vi "1 - Get XY and start end.vi"() -> ()   [LabVIEW 2013]
uses:
  <vilib>/vision/NI_Vision_Development_Module.lvlib
panel:
  out "appended array":dbl[](array[numeric])
  out "frame number XY top XY bottom":dbl[][](array[numeric])
  in  "fast forward":bool
  out "start":i32[](array[numeric])
  out "end":i32[](array[numeric])
  out "end":i32[](array[numeric])
  out "start":i32[](array[numeric])
  in  "start":bool
  in  "End":bool
  out "Number of Frames":u32
  out "Top VIew":cluster{"Numeric":dbl, "Numeric":dbl}[](graph)
  out "Image 4":T1(plugin-control)
  in  "frame jump":i32=3
  in  "speed":u32(slide)
  in  "start":i32(slide) step=219843704 scale=0.0..44796.0
  out "Image 3":T1(plugin-control)
  in  "AVI Path":path=path "E:/PhD work/PhD research work/Videos/Chen Jin vs Hu Yun (Edited).avi"
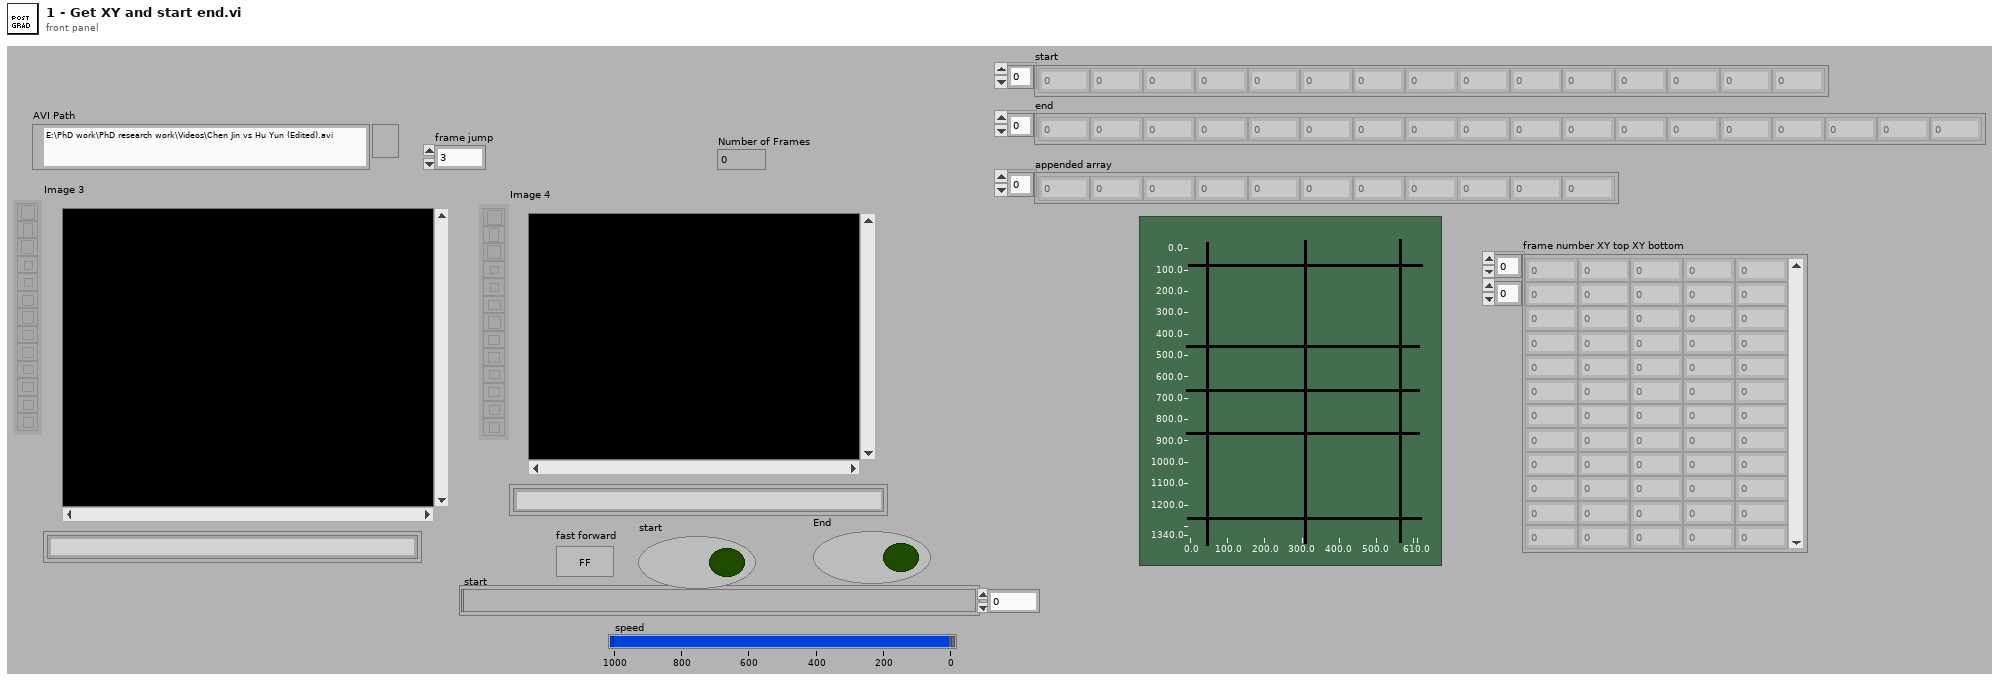
[diagram p1: front panel]
types:
  T1 = typedef "IMAQ Image.ctl" = refnum<image>
  T2 = cluster{cluster{"X":sgl, "Y":sgl}[], cluster{i32, i32}[], "Unit":u32}
  T3 = typedef "Image Type" = u32
  T4 = typedef "AviRefnum.ctl" = refnum<k1>
  T5 = cluster{"width":u32, "height":u32, "framesPerSecond":u32, "compressionFilter":string, "hasData":bool}
  T6 = cluster{"Origin Pixel":cluster{"X":sgl, "Y":sgl}, "Angle Relative to Horizontal (deg)":sgl, "Axis Reference":u32}
  T7 = typedef "Particle Parameters" = i32
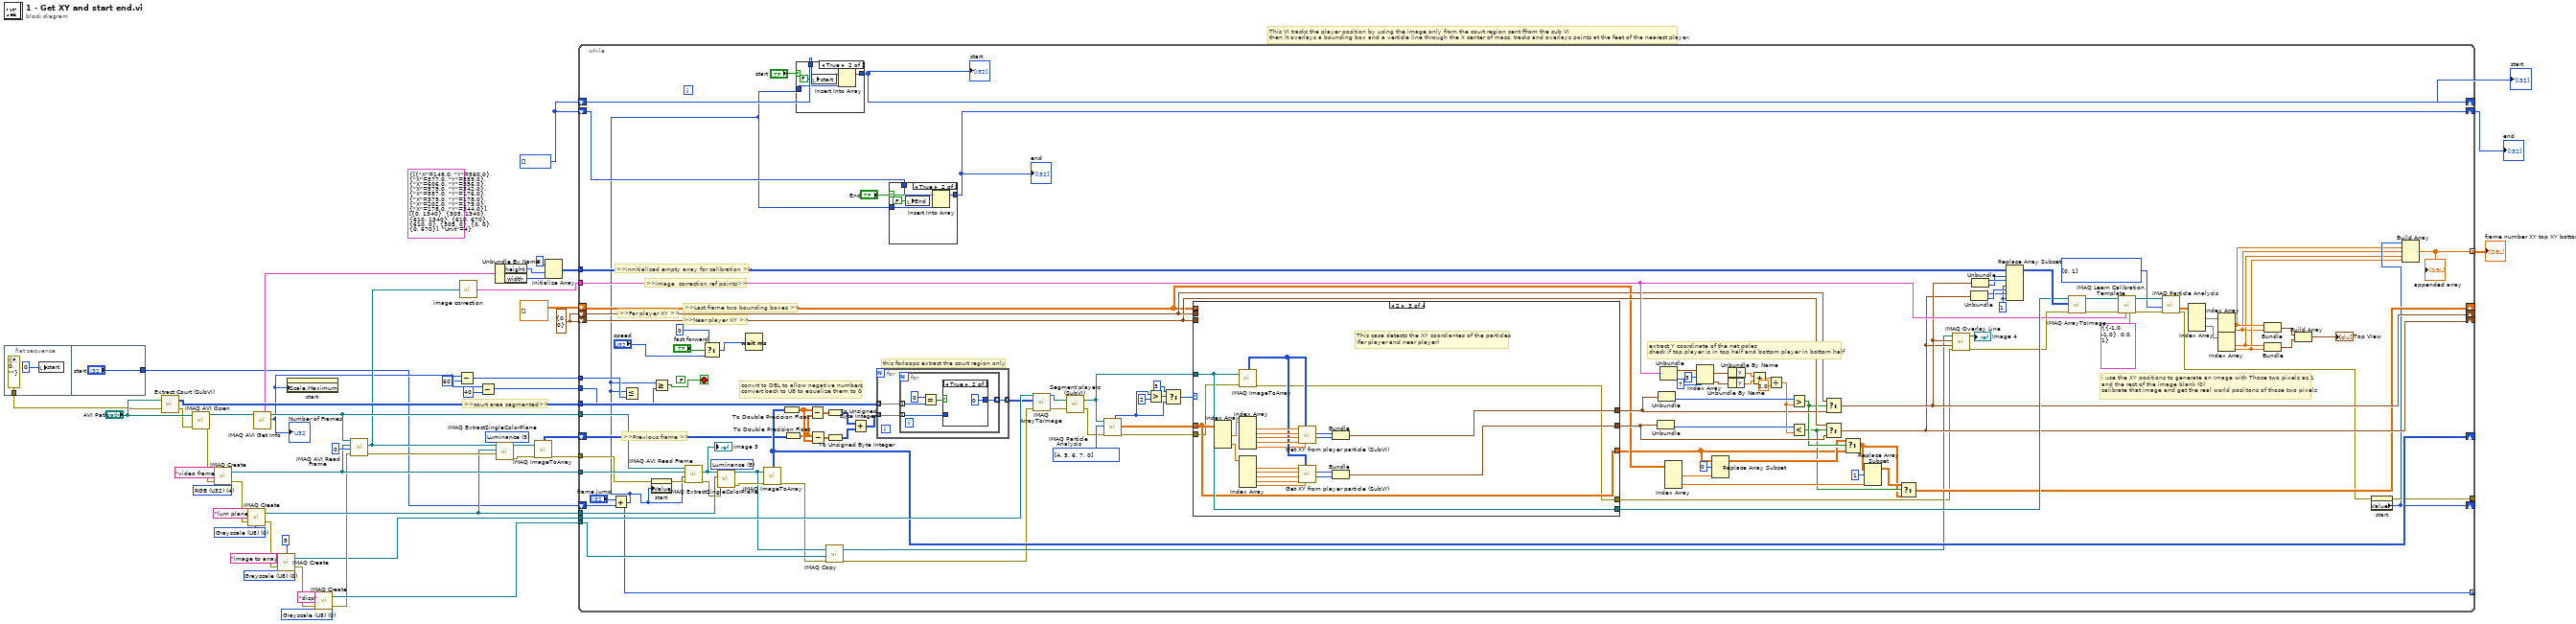
[diagram p0: block diagram]
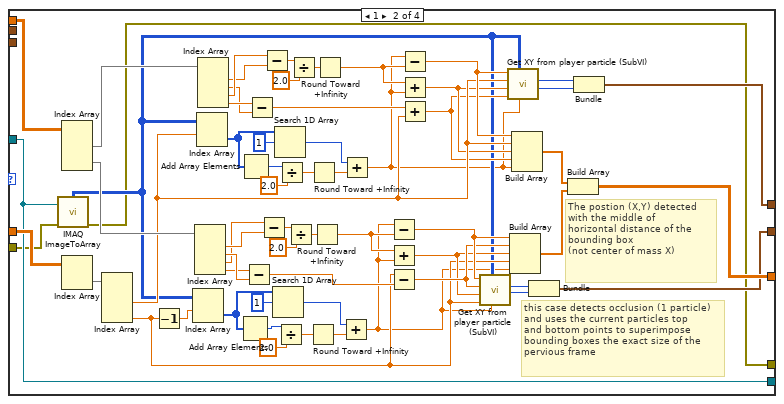
[diagram p5: hidden frame]
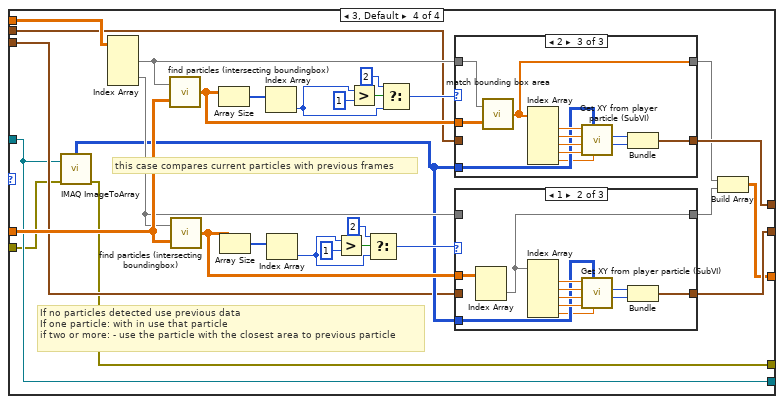
[diagram p6: hidden frame]
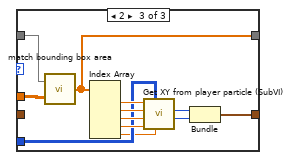
[diagram p8: hidden frame]
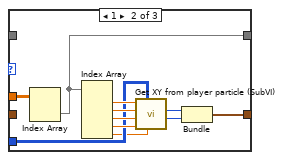
[diagram p10: hidden frame]
diagram:
  (unwired) T2 {[{"X"=148.0, "Y"=560.0}, {"X"=377.0, "Y"=559.0}, {"X"=606.0, "Y"=556.0}, {"X"=579.0, "Y"=342.0}, {"X"=557.0, "Y"=176.0}, {"X"=379.0, "Y"=178.0}, {"X"=202.0, "Y"=179.0}, {"X"=178.0, "Y"=344.0}], [{0, 1340}, {305, 1340}, {610, 1340}, {610, 670}, {610, 0}, {305, 0}, {0, 0}, {0, 670}], "Unit"=4} ("ref points")
  w6 = i32[] [] ("input array")
  w22 = cluster{"X coordinate":i32, "Y coordinate":i32} {"X coordinate"=0, "Y coordinate"=0}
  w35 = T3 0 items=["Grayscale (U8)", "Grayscale (I16)", "Grayscale (SGL)", "Complex (CSG)", "RGB (U32)", "HSL (U32)", "RGB (U64)", "Grayscale (U16)"] ("Image Type")
  w42 = 5 items=["Red", "Green", "Blue", "Hue", "Saturation", "Luminance", "Value", "Intensity"] ("Color Plane")
  w43 = T3 0 items=["Grayscale (U8)", "Grayscale (I16)", "Grayscale (SGL)", "Complex (CSG)", "RGB (U32)", "HSL (U32)", "RGB (U64)", "Grayscale (U16)"] ("Image Type")
  w47 = T3 0 items=["Grayscale (U8)", "Grayscale (I16)", "Grayscale (SGL)", "Complex (CSG)", "RGB (U32)", "HSL (U32)", "RGB (U64)", "Grayscale (U16)"] ("Image Type")
  w45 = T3 4 items=["Grayscale (U8)", "Grayscale (I16)", "Grayscale (SGL)", "Complex (CSG)", "RGB (U32)", "HSL (U32)", "RGB (U64)", "Grayscale (U16)"] ("Image Type")
  # ">>court area segmented>>"
  # "This VI tracks the player position by using the image only from the court region sent ffrom the sub VI\nthen it overlays a bounding box and a verticle line through the X center of mass. tracks and overlays points at the feet of the nearest player."
  n1 = flat-sequence {
    tunnel: [errorcluster {"status"=FALSE, "code"=0, "source"=""} ("error in (no error)")] -> w3
    tunnel: ["start"] -> w1
    frame #0 {
      n2 = local write "start"(0 ("start")) -> ()
    }
    frame #1 {
    }
  }
  n3 = call "Extract Court (SubVI).vi"("error in (no error)"=w3, "AVI Path"="AVI Path") -> ("error out"=w49:errorcluster, "Court pixels out"=w25:u8[][])
  n4 = call "IMAQ AVI Open"("error in (no error)"=w49, "AVI Path"="AVI Path") -> ("error out"=w31:errorcluster, "Avi Refnum"=w21:T4)  [unwired: 8 in]
  n5 = call "IMAQ Create"("Image Name"="video frame", "Image Type"=w45, "error in (no error)"=w31) -> ("New Image"=w39:T1, "error out"=w30:errorcluster)  [unwired: 2 in]
  n6 = call "IMAQ Create"("Image Name"="lum plane", "Image Type"=w47, "error in (no error)"=w30) -> ("New Image"=w38:T1, "error out"=w29:errorcluster)  [unwired: 2 in]
  n7 = call "IMAQ AVI Get Info"("Avi Refnum"=w21) -> ("Number of Frames"=w12:u32, "Avi Refnum (duplicate)"=w20:T4, "Frame Data"=w17:T5)  [unwired: 6 in, 2 out]
  "Number of Frames" <- w12
  n8 = call "IMAQ Create"("Border Size"=5, "Image Name"="image to array", "Image Type"=w43, "error in (no error)"=w29) -> ("New Image"=w24:T1, "error out"=w28:errorcluster)  [unwired: 1 in]
  n9 = property on="start" class="Slide (strict)"("Scale.Maximum"=w12) -> ()  [unwired: 2 in, 2 out]
  n10 = call "IMAQ Create"("Image Name"="disp", "Image Type"=w35, "error in (no error)"=w28) -> ("New Image"=w33:T1, "error out"=w27:errorcluster)  [unwired: 2 in]
  n11 = call "IMAQ AVI Read Frame"("error in (no error)"=w27, "Frame Number"=u32 0, "Image"=w39, "Avi Refnum"=w20) -> ("error out"=w41:errorcluster, "Image Out"=w13:T1)  [unwired: 4 in, 2 out]
  n12 = Subtract(x=w12, y=u32 60) -> (x-y=w9:u32)
  n13 = call "image correction.vi"("Image"=w13) -> ("ref points"=w7:T2)
  n14 = Subtract(x=w12, y=u32 40) -> (x-y=w8:u32)
  n15 = Unbundle By Name(w17) -> ("height"=w16:u32, "width"=w15:u32)
  n16 = call "IMAQ ExtractSingleColorPlane"("Color Plane"=w42, "error in (no error)"=w41, "Image Dst"=w38, "Image Src"=w13) -> ("error out"=w32:errorcluster, "Image Dst Out"=w36:T1)  [unwired: 6 in]
  n17 = call "IMAQ ImageToArray"("error in (no error)"=w32, "Image"=w36) -> ("error out"=w19:errorcluster, "Image Pixels (U8)"=w37:u8[][])  [unwired: 2 in, 3 out]
  n18 = Initialize Array(u8 0 ("element"), w16, w15) -> (w14:u8[][])
  n19 = while {
    tunnel: w20 -> [w138]
    tunnel: w39 -> [w155]
    tunnel: w25 -> [w168]
    tunnel: w38 -> [w156]
    tunnel: w24 -> [w167]
    shift-right: [w166] -> _
    shift-left: w37 -> [w165]
    tunnel: w33 -> [w141]
    shift-right: [w88] -> _
    shift-left: dbl[][] [] ("Particle Measurements (Pixels)") -> [w98]
    shift-right: [w102] -> _
    shift-left: w22 -> [w104]
    shift-right: [w100] -> _
    shift-left: w22 -> [w103]
    shift-right: [w60] -> _
    shift-left: w1 -> [w140]
    tunnel: w19 -> [w137]
    tunnel: w14 -> [w135]
    tunnel: w7 -> [w117]
    tunnel: [w80] -> _
    tunnel: w9 -> [w78]
    tunnel: w8 -> [w77]
    tunnel: [w54] -> _ mode=indexing
    shift-right: [w68] -> w4
    shift-left: w6 -> [w69]
    shift-right: [w70] -> w5
    shift-left: w6 -> [w71]
    tunnel: [w56] -> w2 mode=indexing
    stop <- w79 stop-if-true
    w122 = T7[] [0, 1] items=["Center of Mass X", "Center of Mass Y", "First Pixel X", "First Pixel Y", "Bounding Rect Left", "Bounding Rect Top", "Bounding Rect Right", "Bounding Rect Bottom", "Max Feret Diameter Start X", "Max Feret Diameter Start Y", "Max Feret Diameter End X", "Max Feret Diameter End Y", "Max Horiz. Segment Length Left", "Max Horiz. Segment Length Right", "Max Horiz. Segment Length Row", "-", "Bounding Rect Width", "Bounding Rect Height", "Bounding Rect Diagonal", "Perimeter", "Convex Hull Perimeter", "Holes' Perimeter", "Max Feret Diameter", "Equivalent Ellipse Major Axis", "Equivalent Ellipse Minor Axis", "Equivalent Ellipse Minor Axis (Feret)", "Equivalent Rect Long Side", "Equivalent Rect Short Side", "Equivalent Rect Diagonal", "Equivalent Rect Short Side (Feret)", "Average Horiz. Segment Length", "Average Vert. Segment Length", "Hydraulic Radius", "Waddel Disk Diameter", "-", "Area", "Holes' Area", "Particle & Holes' Area", "Convex Hull Area", "Image Area", "-", "Number of Holes", "Number of Horiz. Segments", "Number of Vert. Segments", "-", "Orientation", "Max Feret Diameter Orientation", "-", "% Area/Image Area", "% Area/(Particle & Holes' Area)", "Ratio of Equivalent Ellipse Axes", "Ratio of Equivalent Rect Sides", "-", "Elongation Factor", "Compactness Factor", "Heywood Circularity Factor", "Type Factor", "-", "Sum X", "Sum Y", "Sum XX", "Sum XY", "Sum YY", "Sum XXX", "Sum XXY", "Sum XYY", "Sum YYY", "-", "Moment of Inertia XX", "Moment of Inertia XY", "Moment of Inertia YY", "Moment of Inertia XXX", "Moment of Inertia XXY", "Moment of Inertia XYY", "Moment of Inertia YYY", "Norm. Moment of Inertia XX", "Norm. Moment of Inertia XY", "Norm. Moment of Inertia YY", "Norm. Moment of Inertia XXX", "Norm. Moment of Inertia XXY", "Norm. Moment of Inertia XYY", "Norm. Moment of Inertia YYY", "Hu Moment 1", "Hu Moment 2", "Hu Moment 3", "Hu Moment 4", "Hu Moment 5", "Hu Moment 6", "Hu Moment 7"] ("Real-World Measurements")
    w130 = u8 1 ("new element/subarray")
    w157 = T7[] [4, 5, 6, 7, 0] items=["Center of Mass X", "Center of Mass Y", "First Pixel X", "First Pixel Y", "Bounding Rect Left", "Bounding Rect Top", "Bounding Rect Right", "Bounding Rect Bottom", "Max Feret Diameter Start X", "Max Feret Diameter Start Y", "Max Feret Diameter End X", "Max Feret Diameter End Y", "Max Horiz. Segment Length Left", "Max Horiz. Segment Length Right", "Max Horiz. Segment Length Row", "-", "Bounding Rect Width", "Bounding Rect Height", "Bounding Rect Diagonal", "Perimeter", "Convex Hull Perimeter", "Holes' Perimeter", "Max Feret Diameter", "Equivalent Ellipse Major Axis", "Equivalent Ellipse Minor Axis", "Equivalent Ellipse Minor Axis (Feret)", "Equivalent Rect Long Side", "Equivalent Rect Short Side", "Equivalent Rect Diagonal", "Equivalent Rect Short Side (Feret)", "Average Horiz. Segment Length", "Average Vert. Segment Length", "Hydraulic Radius", "Waddel Disk Diameter", "-", "Area", "Holes' Area", "Particle & Holes' Area", "Convex Hull Area", "Image Area", "-", "Number of Holes", "Number of Horiz. Segments", "Number of Vert. Segments", "-", "Orientation", "Max Feret Diameter Orientation", "-", "% Area/Image Area", "% Area/(Particle & Holes' Area)", "Ratio of Equivalent Ellipse Axes", "Ratio of Equivalent Rect Sides", "-", "Elongation Factor", "Compactness Factor", "Heywood Circularity Factor", "Type Factor", "-", "Sum X", "Sum Y", "Sum XX", "Sum XY", "Sum YY", "Sum XXX", "Sum XXY", "Sum XYY", "Sum YYY", "-", "Moment of Inertia XX", "Moment of Inertia XY", "Moment of Inertia YY", "Moment of Inertia XXX", "Moment of Inertia XXY", "Moment of Inertia XYY", "Moment of Inertia YYY", "Norm. Moment of Inertia XX", "Norm. Moment of Inertia XY", "Norm. Moment of Inertia YY", "Norm. Moment of Inertia XXX", "Norm. Moment of Inertia XXY", "Norm. Moment of Inertia XYY", "Norm. Moment of Inertia YYY", "Hu Moment 1", "Hu Moment 2", "Hu Moment 3", "Hu Moment 4", "Hu Moment 5", "Hu Moment 6", "Hu Moment 7"] ("Pixel Measurements")
    (unwired) FALSE
    w169 = 5 items=["Red", "Green", "Blue", "Hue", "Saturation", "Luminance", "Value", "Intensity"] ("Color Plane")
    # ">>innitialized empty array for calibration >>"
    # ">>image  correction ref points>>"
    # "extract Y coordinate of the net poles\ncheck if top player is in top half and bottom player in bottom half"
    # "i use the XY positions to generate an Image with Those two pixels as 1 \nand the rest of the image blank (0)\ncalibrate that image and get the real world posiitons of those two pixels"
    # ">>Last frame two bounding boxes >>"
    # ">>Far player XY >>"
    # ">>Near player XY >>"
    # ">>Previous frame >>"
    # "convrt to DBL to allow negative numbers\nconvert back to U8 to equalize them to 0"
    # "this forloops extract the court region only"
    n20 = Add(x="frame jump", y=w140) -> (x+y=w54:i32)
    n21 = Less Or Equal?(x=w54, y=w78) -> ()  [unwired: 1 out]
    n22 = property on="start" class="Slide (strict)"(error in=w137, "Value"=w54) -> (error out=w136:errorcluster)  [unwired: 1 in, 1 out]
    n23 = Greater Or Equal?(x=w54, y=w77) -> (x >= y?=w79:bool)
    n24 = call "IMAQ AVI Read Frame"("error in (no error)"=w136, "Frame Number"=w54, "Image"=w155, "Avi Refnum"=w138) -> ("error out"=w73:errorcluster, "Image Out"=w76:T1)  [unwired: 4 in, 2 out]
    "Image 3" <- w76
    n25 = Select(t=u32 0, s="fast forward", f="speed") -> (s? t:f=w62:u32)
    n26 = call "IMAQ ExtractSingleColorPlane"("Color Plane"=w169, "error in (no error)"=w73, "Image Dst"=w156, "Image Src"=w76) -> ("error out"=w158:errorcluster, "Image Dst Out"=w142:T1)  [unwired: 6 in]
    n27 = Wait (ms)(milliseconds to wait=w62) -> ()  [unwired: 1 out]
    n28 = call "IMAQ ImageToArray"("error in (no error)"=w158, "Image"=w142) -> ("error out"=w85:errorcluster, "Image Pixels (U8)"=w166:u8[][])  [unwired: 2 in, 3 out]
    n29 = To Double Precision Float(number=w166) -> (double precision float=w162:dbl[][])
    n30 = To Double Precision Float(number=w165) -> (double precision float=w161:dbl[][])
    n31 = case shown="True" "start" {
      tunnel: w71 -> [w175 w179]
      tunnel: w54 -> [_ w178]
      tunnel: [w175 w177] -> w70
      frame False {
      }
      frame True {
        n32 = local write "start"(FALSE ("start")) -> ()
        n33 = Insert Into Array(array=w179, new element=w178) -> (w177:i32[])  [unwired: 1 in]
      }
    }
    "start" <- w70
    n34 = Subtract(x=w162, y=w161) -> (x-y=w160:dbl[][])
    n35 = Subtract(x=w161, y=w162) -> (x-y=w159:dbl[][])
    n36 = call "IMAQ Copy"("error in (no error)"=w85, "Image Dst"=w141, "Image Src"=w142) -> ("error out"=w84:errorcluster, "Image Dst Out"=w86:T1)  [unwired: 3 in]
    n37 = To Unsigned Byte Integer(number=w160) -> (unsigned 8bit integer=w164:u8[][])
    n38 = To Unsigned Byte Integer(number=w159) -> (unsigned 8bit integer=w163:u8[][])
    n39 = Add(x=w164, y=w163) -> (x+y=w66:u8[][])
    n40 = for {
      tunnel: w168 -> [w350] mode=indexing
      tunnel: [w349] -> w65 mode=indexing
      tunnel: w66 -> [w348] mode=indexing
      n41 = for {
        tunnel: w350 -> [w355] mode=indexing
        tunnel: [w352] -> w349 mode=indexing
        tunnel: w348 -> [w351] mode=indexing
        n42 = Equal?(x=u8 0, y=w355) -> (x = y?=w353:bool)
        n43 = case shown="True" w353 {
          tunnel: [w356 u8 0 ("x")] -> w352
          tunnel: w351 -> [w356 _]
          frame False {
          }
          frame True {
          }
        }
      }
    }
    n44 = case shown="True" "End" {
      tunnel: w69 -> [w170 w174]
      tunnel: w54 -> [_ w173]
      tunnel: [w170 w172] -> w68
      frame False {
      }
      frame True {
        n45 = local write "End"(FALSE ("End")) -> ()
        n46 = Insert Into Array(array=w174, new element=w173) -> (w172:i32[])  [unwired: 1 in]
      }
    }
    "end" <- w68
    n47 = call "IMAQ ArrayToImage"("error in (no error)"=w84, "Image Pixels (U8)"=w65, "Image"=w167) -> ("error out"=w153:errorcluster, "Image Out"=w154:T1)  [unwired: 7 in]
    n48 = call "Segment players (SubVI).vi"("error In"=w153, "Image In"=w154) -> ("error out"=w147:errorcluster, "Image Out"=w145:T1)
    n49 = call "IMAQ Particle Analysis"("error in (no error)"=w147, "Pixel Measurements"=w157, "Image"=w145) -> ("error out"=w146:errorcluster, "Particle Measurements (Pixels)"=w144:dbl[][], "Number of Particles"=w149:i32)  [unwired: 3 in, 3 out]
    n50 = Greater?(x=w149, y=2) -> (0:w152:bool)
    n51 = Select(t=3 ("y"), s=w152, f=w149) -> (s? t:f=w148:i32)
    n52 = case shown="2" w148 {
      tunnel: [w183 w210 w264 w274] -> w128
      tunnel: w144 -> [_ w245 w250 w294]
      tunnel: w146 -> [w180 w186 w247 w270]
      tunnel: w145 -> [w183 w210 w264 w274]
      tunnel: [w181 w194 w252 w276] -> w99
      tunnel: [w182 w201 w251 w275] -> w101
      tunnel: [w184 w211 w250 w271] -> w87
      tunnel: w98 -> [w184 w235 _ w297]
      tunnel: w104 -> [w182 _ _ w282]
      tunnel: w103 -> [w181 _ _ w277]
      tunnel: [w180 w185 w246 w269] -> w82
      frame 0 {
        # "This case identifies frames where no particles are detected and keeps the same values from the\nprevious frame"
      }
      frame 1 {
        # "The postion (X,Y) detected with the middle of \nhorizontal distance of the bounding box\n(not center of mass X)"
        # "this case detects occlusion (1 particle)\nand uses the current particles top \nand bottom points to superimpose \nbounding boxes the exact size of the \npervious frame"
        n53 = call "IMAQ ImageToArray"("error in (no error)"=w186, "Image"=w210) -> ("error out"=w185:errorcluster, "Image Pixels (U8)"=w193:u8[][])  [unwired: 2 in, 3 out]
        n54 = Index Array(array=w235) -> (element #1=w243:dbl[], element #2=w215:dbl[])  [unwired: 4 in]
        n55 = Index Array(array=w245) -> (element=w244:dbl[])  [unwired: 2 in]
        n56 = Index Array(array=w244) -> (element #2=w206:dbl, element #4=w197:dbl)  [unwired: 4 in, 2 out]
        n57 = Decrement(x=w197) -> (x-1=w208:dbl)
        n58 = Index Array(array=w193, index (row)=w208) -> (element=w230:u8[])  [unwired: 1 in]
        n59 = Index Array(array=w215) -> (element #1=w219:dbl, element #2=w222:dbl, element #3=w218:dbl, element #4=w221:dbl)  [unwired: 4 in]
        n60 = Index Array(array=w193, index (row)=w206) -> (element=w223:u8[])  [unwired: 1 in]
        n61 = Index Array(array=w243) -> (element #1=w239:dbl, element #2=w236:dbl, element #3=w240:dbl, element #4=w237:dbl)  [unwired: 4 in]
        n62 = Add Array Elements(numeric array=w230) -> (sum=w231:u8)
        n63 = Add Array Elements(numeric array=w223) -> (sum=w227:u8)
        n64 = Subtract(x=w221, y=w222) -> (x-y=w209:dbl)
        n65 = Subtract(x=w237, y=w236) -> (x-y=w214:dbl)
        n66 = Subtract(x=w218, y=w219) -> (x-y=w217:dbl)
        n67 = Subtract(x=w240, y=w239) -> (x-y=w241:dbl)
        n68 = Search 1D Array(1D array=w230, element=u8 1) -> (index of element=w229:i32)  [unwired: 1 in]
        n69 = Search 1D Array(1D array=w223, element=u8 1) -> (index of element=w228:i32)  [unwired: 1 in]
        n70 = Divide(x=w231, y=2.0) -> (x/y=w232:dbl)
        n71 = Divide(x=w227, y=2.0) -> (x/y=w226:dbl)
        n72 = Divide(x=w217, y=2.0) -> (x/y=w220:dbl)
        n73 = Divide(x=w241, y=2.0) -> (x/y=w238:dbl)
        n74 = Round Toward +Infinity(x=w232) -> (ceil(x): smallest int >= x=w191:dbl)
        n75 = Round Toward +Infinity(x=w226) -> (ceil(x): smallest int >= x=w190:dbl)
        n76 = Round Toward +Infinity(x=w220) -> (ceil(x): smallest int >= x=w192:dbl)
        n77 = Round Toward +Infinity(x=w238) -> (ceil(x): smallest int >= x=w189:dbl)
        n78 = Add(x=w229, y=w191) -> (x+y=w187:dbl)
        n79 = Add(x=w228, y=w190) -> (x+y=w188:dbl)
        n80 = Subtract(x=w187, y=w192) -> (x-y=w200:dbl)
        n81 = Add(x=w192, y=w187) -> (x+y=w198:dbl)
        n82 = Subtract(x=w197, y=w209) -> (x-y=w199:dbl)
        n83 = Subtract(x=w188, y=w189) -> (x-y=w207:dbl)
        n84 = Add(x=w189, y=w188) -> (x+y=w205:dbl)
        n85 = Add(x=w214, y=w206) -> (x+y=w204:dbl)
        n86 = call "Get XY from player particle (SubVI).vi"("Center of mass X"=w187, "Image in Pixels (U8)"=w193, "Particle bounding rect bottom"=w197, "Particle bounding rect right"=w198, "Particle bounding rect top"=w199, "Particle bounding rect left"=w200) -> ("Y coordinate"=w195:i32, "X coordinate"=w196:i32)  [unwired: 2 in]
        n87 = call "Get XY from player particle (SubVI).vi"("Center of mass X"=w188, "Image in Pixels (U8)"=w193, "Particle bounding rect bottom"=w204, "Particle bounding rect right"=w205, "Particle bounding rect top"=w206, "Particle bounding rect left"=w207) -> ("Y coordinate"=w202:i32, "X coordinate"=w203:i32)  [unwired: 2 in]
        n88 = Build Array(w200, w199, w198, w197, w187) -> (w212:dbl[])
        n89 = Build Array(w207, w206, w205, w204, w188) -> (w213:dbl[])
        n90 = Bundle("X coordinate"=w196, "Y coordinate"=w195) -> (w194:cluster{"X coordinate":i32, "Y coordinate":i32})  [unwired: 1 in]
        n91 = Build Array(w213, w212) -> (w211:dbl[][])
        n92 = Bundle("X coordinate"=w203, "Y coordinate"=w202) -> (w201:cluster{"X coordinate":i32, "Y coordinate":i32})  [unwired: 1 in]
      }
      frame 2 {
        # "This case detects the XY coordiantes of the particles\n(far player and near player)"
        n93 = Index Array(array=w250) -> (element #1=w258:dbl[], element #2=w257:dbl[])  [unwired: 4 in]
        n94 = call "IMAQ ImageToArray"("error in (no error)"=w247, "Image"=w264) -> ("error out"=w246:errorcluster, "Image Pixels (U8)"=w259:u8[][])  [unwired: 2 in, 3 out]
        n95 = Index Array(array=w258) -> (element #1=w268:dbl, element #2=w267:dbl, element #3=w266:dbl, element #4=w265:dbl, element #5=w249:dbl)  [unwired: 5 in]
        n96 = Index Array(array=w257) -> (element #1=w260:dbl, element #2=w261:dbl, element #3=w262:dbl, element #4=w263:dbl, element #5=w248:dbl)  [unwired: 5 in]
        n97 = call "Get XY from player particle (SubVI).vi"("Center of mass X"=w249, "Image in Pixels (U8)"=w259, "Particle bounding rect bottom"=w265, "Particle bounding rect right"=w266, "Particle bounding rect top"=w267, "Particle bounding rect left"=w268) -> ("Y coordinate"=w255:i32, "X coordinate"=w256:i32)  [unwired: 2 in]
        n98 = call "Get XY from player particle (SubVI).vi"("Center of mass X"=w248, "Image in Pixels (U8)"=w259, "Particle bounding rect bottom"=w263, "Particle bounding rect right"=w262, "Particle bounding rect top"=w261, "Particle bounding rect left"=w260) -> ("Y coordinate"=w253:i32, "X coordinate"=w254:i32)  [unwired: 2 in]
        n99 = Bundle("X coordinate"=w256, "Y coordinate"=w255) -> (w251:cluster{"X coordinate":i32, "Y coordinate":i32})  [unwired: 1 in]
        n100 = Bundle("X coordinate"=w254, "Y coordinate"=w253) -> (w252:cluster{"X coordinate":i32, "Y coordinate":i32})  [unwired: 1 in]
      }
      frame 3, Default {
        # "If no particles detected use previous data\nIf one particle: with in use that particle\nif two or more: - use the particle with the closest area to previous particle"
        # "this case compares current particles with previous frames"
        n101 = call "IMAQ ImageToArray"("error in (no error)"=w270, "Image"=w274) -> ("error out"=w269:errorcluster, "Image Pixels (U8)"=w278:u8[][])  [unwired: 2 in, 3 out]
        n102 = Index Array(array=w297) -> (element #1=w293:dbl[], element #2=w281:dbl[])  [unwired: 4 in]
        n103 = call "find particles (intersecting boundingbox).vi"("Particle Measurements in (bounding boxes)"=w294, "bounding box in"=w293) -> ("Particles within bounding box"=w292:dbl[][])
        n104 = call "find particles (intersecting boundingbox).vi"("Particle Measurements in (bounding boxes)"=w294, "bounding box in"=w281) -> ("Particles within bounding box"=w279:dbl[][])
        n105 = Array Size(array=w292) -> (size(s)=w296:i32[])
        n106 = Array Size(array=w279) -> (size(s)=w295:i32[])
        n107 = Index Array(array=w296) -> (element=w284:i32)  [unwired: 1 in]
        n108 = Index Array(array=w295) -> (element=w285:i32)  [unwired: 1 in]
        n109 = Greater?(x=w285, y=1) -> (0:w288:bool)
        n110 = Greater?(x=w284, y=1) -> (0:w289:bool)
        n111 = Select(t=2 ("y"), s=w288, f=w285) -> (s? t:f=w280:i32)
        n112 = Select(t=2 ("y"), s=w289, f=w284) -> (s? t:f=w283:i32)
        n113 = case shown="2" w283 {
          tunnel: w293 -> [w324 _ w339]
          tunnel: w292 -> [_ w335 w338]
          tunnel: [w324 w326 w337] -> w273
          tunnel: w278 -> [_ w328 w341]
          tunnel: [w323 w327 w340] -> w275
          tunnel: w282 -> [w323 _ _]
          frame 0, Default {
          }
          frame 1 {
            n114 = Index Array(array=w335) -> (element=w326:dbl[])  [unwired: 2 in]
            n115 = Index Array(array=w326) -> (element #1=w332:dbl, element #2=w331:dbl, element #3=w330:dbl, element #4=w329:dbl, element #5=w325:dbl)  [unwired: 5 in]
            n116 = call "Get XY from player particle (SubVI).vi"("Center of mass X"=w325, "Image in Pixels (U8)"=w328, "Particle bounding rect bottom"=w329, "Particle bounding rect right"=w330, "Particle bounding rect top"=w331, "Particle bounding rect left"=w332) -> ("Y coordinate"=w333:i32, "X coordinate"=w334:i32)  [unwired: 2 in]
            n117 = Bundle("X coordinate"=w334, "Y coordinate"=w333) -> (w327:cluster{"X coordinate":i32, "Y coordinate":i32})  [unwired: 1 in]
          }
          frame 2 {
            n118 = call "match bounding box area.vi"("particle measurements (bounding box)"=w338, "bounding box in"=w339) -> ("matching bounding box"=w337:dbl[])
            n119 = Index Array(array=w337) -> (element #1=w345:dbl, element #2=w344:dbl, element #3=w343:dbl, element #4=w342:dbl, element #5=w336:dbl)  [unwired: 5 in]
            n120 = call "Get XY from player particle (SubVI).vi"("Center of mass X"=w336, "Image in Pixels (U8)"=w341, "Particle bounding rect bottom"=w342, "Particle bounding rect right"=w343, "Particle bounding rect top"=w344, "Particle bounding rect left"=w345) -> ("Y coordinate"=w346:i32, "X coordinate"=w347:i32)  [unwired: 2 in]
            n121 = Bundle("X coordinate"=w347, "Y coordinate"=w346) -> (w340:cluster{"X coordinate":i32, "Y coordinate":i32})  [unwired: 1 in]
          }
        }
        n122 = case shown="1" w280 {
          tunnel: w281 -> [w299 _ w314]
          tunnel: w279 -> [_ w310 w313]
          tunnel: [w299 w301 w312] -> w272
          tunnel: w278 -> [_ w303 w316]
          tunnel: [w298 w302 w315] -> w276
          tunnel: w277 -> [w298 _ _]
          frame 0, Default {
          }
          frame 1 {
            n123 = Index Array(array=w310) -> (element=w301:dbl[])  [unwired: 2 in]
            n124 = Index Array(array=w301) -> (element #1=w307:dbl, element #2=w306:dbl, element #3=w305:dbl, element #4=w304:dbl, element #5=w300:dbl)  [unwired: 5 in]
            n125 = call "Get XY from player particle (SubVI).vi"("Center of mass X"=w300, "Image in Pixels (U8)"=w303, "Particle bounding rect bottom"=w304, "Particle bounding rect right"=w305, "Particle bounding rect top"=w306, "Particle bounding rect left"=w307) -> ("Y coordinate"=w308:i32, "X coordinate"=w309:i32)  [unwired: 2 in]
            n126 = Bundle("X coordinate"=w309, "Y coordinate"=w308) -> (w302:cluster{"X coordinate":i32, "Y coordinate":i32})  [unwired: 1 in]
          }
          frame 2 {
            n127 = call "match bounding box area.vi"("particle measurements (bounding box)"=w313, "bounding box in"=w314) -> ("matching bounding box"=w312:dbl[])
            n128 = Index Array(array=w312) -> (element #1=w320:dbl, element #2=w319:dbl, element #3=w318:dbl, element #4=w317:dbl, element #5=w311:dbl)  [unwired: 5 in]
            n129 = call "Get XY from player particle (SubVI).vi"("Center of mass X"=w311, "Image in Pixels (U8)"=w316, "Particle bounding rect bottom"=w317, "Particle bounding rect right"=w318, "Particle bounding rect top"=w319, "Particle bounding rect left"=w320) -> ("Y coordinate"=w321:i32, "X coordinate"=w322:i32)  [unwired: 2 in]
            n130 = Bundle("X coordinate"=w322, "Y coordinate"=w321) -> (w315:cluster{"X coordinate":i32, "Y coordinate":i32})  [unwired: 1 in]
          }
        }
        n131 = Build Array(w273, w272) -> (w271:dbl[][])
      }
    }
    n132 = Unbundle(w99) -> ("Y coordinate"=w106:i32)  [unwired: 1 out]
    n133 = Unbundle(w101) -> ("Y coordinate"=w107:i32)  [unwired: 1 out]
    n134 = Unbundle(w117) -> (w116:cluster{"X":sgl, "Y":sgl}[])  [unwired: 2 out]
    n135 = Index Array(array=w98) -> (element #1=w96:dbl[], element #2=w92:dbl[])  [unwired: 4 in]
    n136 = Index Array(array=w116, index #1=3 ("index"), index #2=7 ("index")) -> (element #1=w113:cluster{"X":sgl, "Y":sgl}, element #2=w112:cluster{"X":sgl, "Y":sgl})
    n137 = Replace Array Subset(array=w87, new element=w96, index (row)=0) -> (w95:dbl[][])  [unwired: 1 in]
    n138 = Unbundle By Name(w112) -> ("Y"=w110:sgl)
    n139 = Unbundle By Name(w113) -> ("Y"=w111:sgl)
    n140 = Add(x=w111, y=w110) -> (x+y=w109:sgl)
    n141 = Divide(x=w109, y=sgl 2.0) -> (x/y=w105:sgl)
    n142 = Greater?(x=w107, y=w105) -> (0:w97:bool)
    n143 = Less?(x=w106, y=w105) -> (x < y?=w90:bool)
    n144 = Select(t=w104, s=w97, f=w101) -> (s? t:f=w102:cluster{"X coordinate":i32, "Y coordinate":i32})
    n145 = Select(t=w103, s=w90, f=w99) -> (s? t:f=w100:cluster{"X coordinate":i32, "Y coordinate":i32})
    n146 = Select(t=w95, s=w97, f=w87) -> (s? t:f=w89:dbl[][])
    n147 = Replace Array Subset(array=w89, new element=w92, index (row)=1) -> (w91:dbl[][])  [unwired: 1 in]
    n148 = Select(t=w91, s=w90, f=w89) -> (s? t:f=w88:dbl[][])
    n149 = call "IMAQ Overlay Line"("error in (no error)"=w82, "End Point"=w100, "Start Point"=w102, "Image"=w86) -> ("error out"=w83:errorcluster, "Image Out"=→"Image 4":T1)  [unwired: 6 in]
    n150 = Unbundle(w100) -> ("X coordinate"=w131:i32, "Y coordinate"=w132:i32)
    n151 = Unbundle(w102) -> ("X coordinate"=w134:i32, "Y coordinate"=w133:i32)
    n152 = Replace Array Subset(array=w135, new element #1=w130, index (row) #1=w133, index (col) #1=w134, new element #2=w130, index (row) #2=w132, index (col) #2=w131) -> (w129:u8[][])
    n153 = call "IMAQ ArrayToImage"("error in (no error)"=w83, "Image Pixels (U8)"=w129, "Image"=w128) -> ("error out"=w125:errorcluster, "Image Out"=w126:T1)  [unwired: 7 in]
    n154 = call "IMAQ Learn Calibration Template"("Calibration Axis Info"=T6 {"Origin Pixel"={"X"=-1.0, "Y"=-1.0}, "Angle Relative to Horizontal (deg)"=0.0, "Axis Reference"=1}, "Reference Points"=w117, "error in (no error)"=w125, "Image"=w126) -> ("error out"=w124:errorcluster, "Calibrated Image"=w123:T1)  [unwired: 5 in, 1 out]
    n155 = call "IMAQ Particle Analysis"("error in (no error)"=w124, "Real-World Measurements"=w122, "Image"=w123) -> ("error out"=w81:errorcluster, "Particle Measurements (Real-World)"=w121:dbl[][])  [unwired: 3 in, 4 out]
    n156 = Index Array(array=w121) -> (element #1=w120:dbl[], element #2=w119:dbl[])  [unwired: 4 in]
    n157 = Index Array(array=w120) -> (element #1=w59:dbl, element #2=w55:dbl)  [unwired: 2 in]
    n158 = Index Array(array=w119) -> (element #1=w58:dbl, element #2=w57:dbl)  [unwired: 2 in]
    n159 = Bundle("Numeric"=w59, "Numeric"=w55) -> (w118:cluster{"Numeric":dbl, "Numeric":dbl})  [unwired: 1 in]
    n160 = Bundle("Numeric"=w58, "Numeric"=w57) -> (w74:cluster{"Numeric":dbl, "Numeric":dbl})  [unwired: 1 in]
    n161 = Build Array(w118, w74) -> (→"Top VIew":cluster{"Numeric":dbl, "Numeric":dbl}[])
    n162 = property on="start" class="Slide (strict)"(error in=w81) -> (error out=w80:errorcluster, "Value"=w60:i32)  [unwired: 1 in, 1 out]
    n163 = Build Array(w60, w59, w55, w58, w57) -> (w56:dbl[])
    "appended array" <- w56
  }
  "end" <- w4
  "start" <- w5
  "frame number XY top XY bottom" <- w2
